vi "Delayed Output.vi"(1 "Interval (ms)":u32=1000, 2 "Input":bool) -> (0 "Delayed Output":bool)   [LabVIEW 2011]
panel:
  # "Input is:\n    False - outputs false\n    True - outputs false, then true when the specified time has passed"
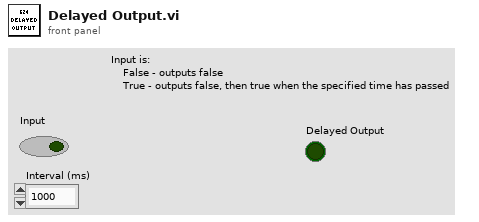
[diagram p1: front panel]
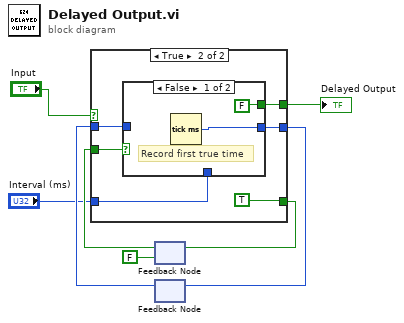
[diagram p0: block diagram]
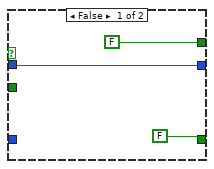
[diagram p2: hidden frame]
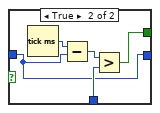
[diagram p3: hidden frame]
diagram:
  n1 = feedback #1(FALSE) -> (w5:bool)
  n2 = feedback #2() -> (w3:u32)  [unwired: 1 in]
  n3 = case shown="True" "Input" {
    tunnel: [FALSE w13] -> w7
    tunnel: [FALSE TRUE] -> w6
    tunnel: w5 -> [_ w16]
    tunnel: [w9 w15] -> w4
    tunnel: w3 -> [w9 w14]
    tunnel: "Interval (ms)" -> [_ w12]
    frame False {
    }
    frame True {
      n4 = case shown="False" w16 {
        tunnel: [w19 w20] -> w15
        tunnel: w14 -> [_ w20]
        tunnel: [FALSE w22] -> w13
        tunnel: w12 -> [_ w21]
        frame False {
          # "Record first true time"
          n5 = Tick Count (ms)() -> (millisecond timer value=w19:u32)
        }
        frame True {
          n6 = Tick Count (ms)() -> (millisecond timer value=w24:u32)
          n7 = Subtract(x=w24, y=w20) -> (x-y=w23:u32)
          n8 = Greater?(x=w23, y=w21) -> (0:w22:bool)
        }
      }
    }
  }
  "Delayed Output" <- w7
  n9 = feedback-in #1(w6) -> ()
  n10 = feedback-in #2(w4) -> ()
